vi "Update_FFID_Bkgnd_info.vi"(1 "Specific Bkgnd Meas?":bool, 2 "c^2 (ppm^2)":dbl[](array[numeric]), 3 "C (ppm)":dbl[](array[numeric])) -> ()   [LabVIEW 2015]
uses:
  Controls/Analysis_info_cluster.ctl
  Controls/Inst_type.ctl
  Controls/Instrument_Array.ctl
  Globals/Meas_global.vi
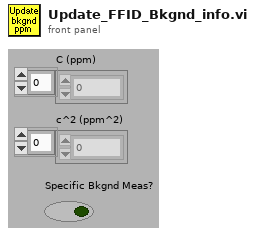
[diagram p1: front panel]
types:
  T1 = cluster{"Weighting":dbl[], "Time (ms)":dbl[], "Voltage":dbl[], "Eng Values":dbl[]}
  T2 = typedef "Analysis_info_cluster.ctl" = cluster{"Colour":u32, "Inst type":T3, "Inst name":string, "Symbol":string, "Code name":string, "Extra Info":string, "Inst Array":T4, "Extra Titles":string[], "Extra Values":string[], "U":dbl, "u^2":dbl, "u^3":dbl, "u^4":dbl, "Skew_u":dbl, "Kurt_u":dbl, "Sd Error in Mean":dbl, "% u'/U":dbl, "X":dbl, "Y":dbl, "Z":dbl, "Timescale integral to 25%":dbl, "Sd Error in Variance":dbl, "Calib File":path, "Calib Constants":dbl[], "Output Position":bool, "Full Stats":bool, "Av Sampling Rate":dbl, "Av No of Samples":dbl, "Total Meas Time (s)":dbl, "ADAM Ch Name":string}
  T3 = typedef "Inst_type.ctl" = enum16{"Propeller anemometer", "Raw voltage", "Pressure Transducer", "Pitot-static tube", "Preston tube", "Hot wire", "Cross wire 1", "Cross wire 2", "Generic Linear", "Generic Polynomial", "Generic BackPoly", "Fast FID", "Thermocouple", "Cold wire", "Pulsed Wire", "LDA Vel", "LDA Tran time", "LDA Arr time", "Microphone"}
  T4 = typedef "Instrument_Array.ctl" = enum16{"PWA", "LDA", "Analogue"}
  T5 = typedef "Time_Trace_Cluster.ctl" = cluster{"Weighting":dbl[], "Time (s)":dbl[], "Voltage":dbl[], "Eng Values":dbl[]}
  T6 = cluster{"Weighting":dbl[], "Time (ms)":dbl[], "Voltage":dbl[], "Eng Values":dbl[]}[]
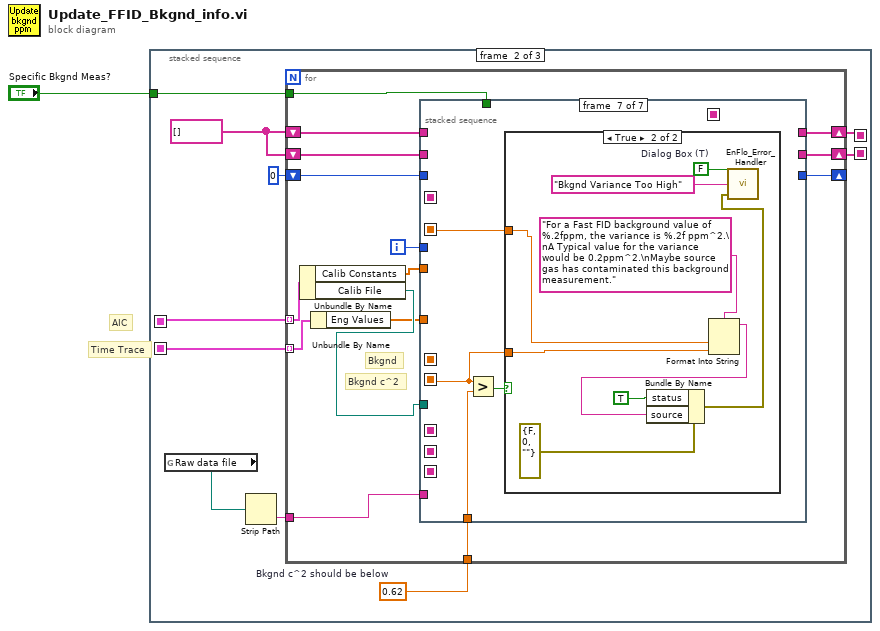
[diagram p0: block diagram]
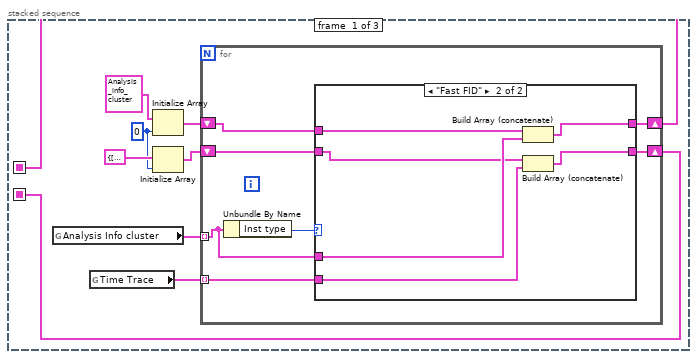
[diagram p2: hidden frame]
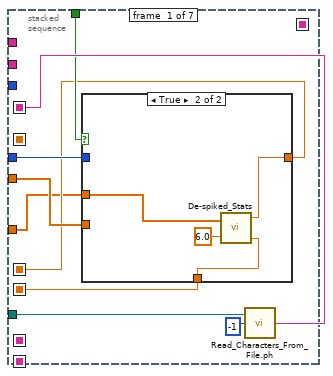
[diagram p4: hidden frame]
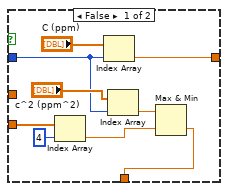
[diagram p5: hidden frame]
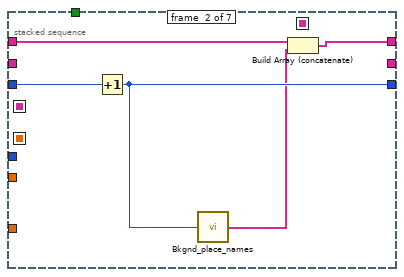
[diagram p6: hidden frame]
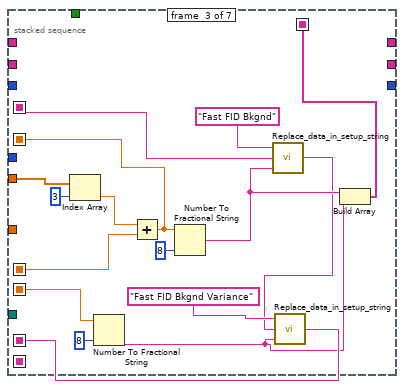
[diagram p7: hidden frame]
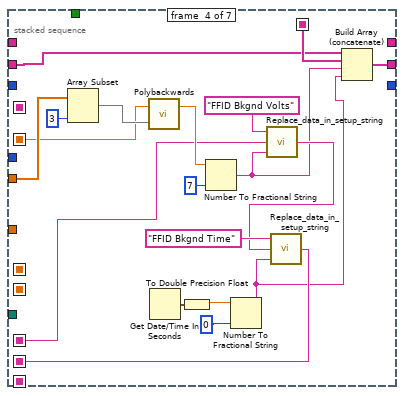
[diagram p8: hidden frame]
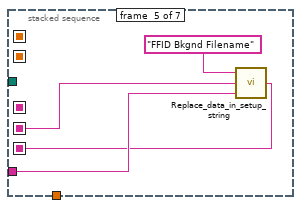
[diagram p9: hidden frame]
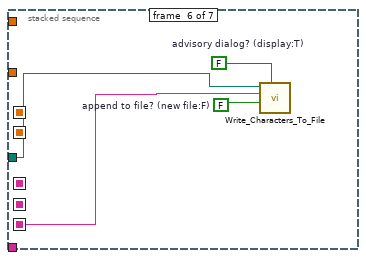
[diagram p10: hidden frame]
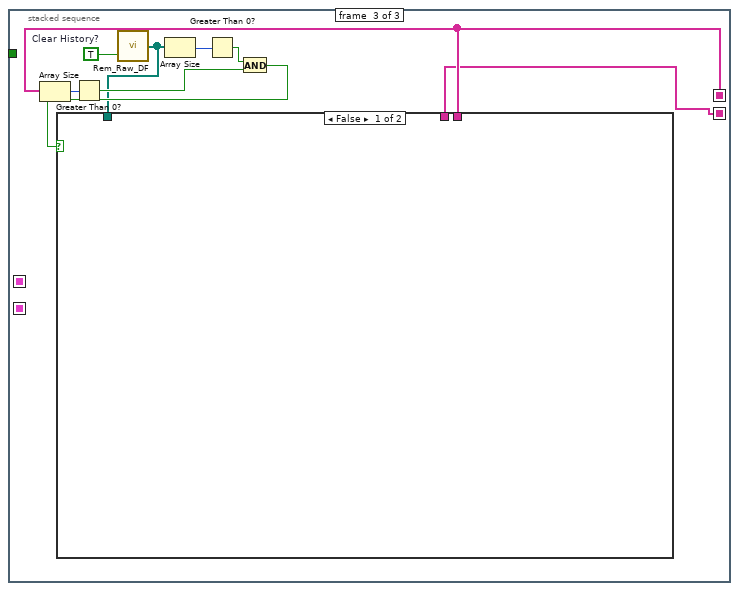
[diagram p12: hidden frame]
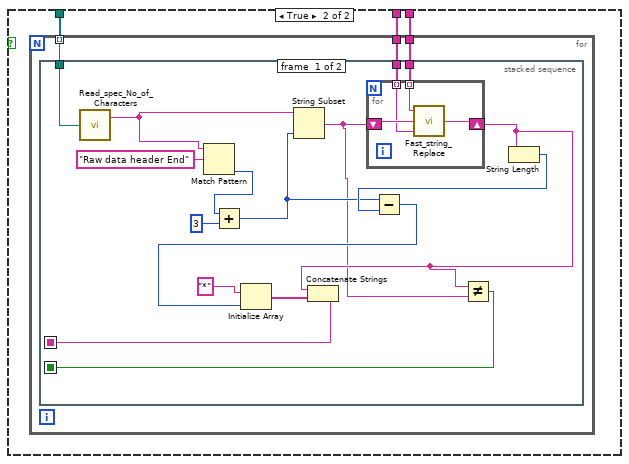
[diagram p13: hidden frame]
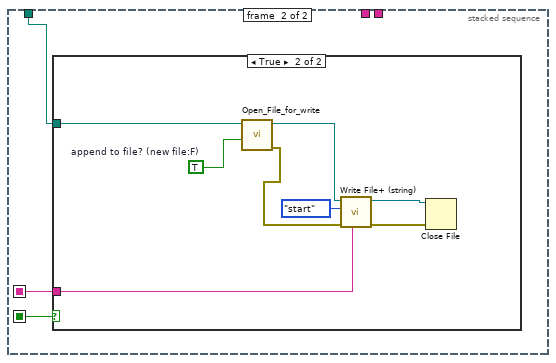
[diagram p14: hidden frame]
diagram:
  # "Time Trace"
  # "AIC"
  n1 = stacked-sequence {
    seq-local: [_ w31 _] -> [_ _ w136]
    seq-local: [_ w30 _] -> [_ _ w135]
    seq-local: [w9 _ _] -> [_ w28 _]
    seq-local: [w2 _ _] -> [_ w26 _]
    tunnel: "Specific Bkgnd Meas?" -> [_ w27 _]
    frame #0 {
      w3 = 0 ("dimension size")
      n2 = global read "Meas_global.vi" "Analysis Info cluster"() -> (w10:T2[])
      n3 = global read "Meas_global.vi" "Time Trace"() -> (w6:T5[])
      n4 = Initialize Array(T2 {"Colour"=0, "Inst type"=enum."Pitot-static tube", "Inst name"="Manometer voltage", "Symbol"="U", "Code name"="", "Extra Info"="U", "Inst Array"=enum."PWA", "Extra Titles"=[], "Extra Values"=[], "U"=0.0, "u^2"=0.0, "u^3"=0.0, "u^4"=0.0, "Skew_u"=0.0, "Kurt_u"=0.0, "Sd Error in Mean"=0.0, "% u'/U"=0.0, "X"=0.0, "Y"=0.0, "Z"=0.0, "Timescale integral to 25%"=0.0, "Sd Error in Variance"=0.0, "Calib File"=path "", "Calib Constants"=[], "Output Position"=FALSE, "Full Stats"=FALSE, "Av Sampling Rate"=0.0, "Av No of Samples"=0.0, "Total Meas Time (s)"=0.0, "ADAM Ch Name"=""} ("Analysis_info_cluster"), w3) -> (w7:T2[])
      n5 = Initialize Array(T1 {"Weighting"=[], "Time (ms)"=[], "Voltage"=[], "Eng Values"=[]} ("Time Trace"), w3) -> (w5:T6)
      n6 = for {
        shift-right: [w15] -> w9
        shift-left: w7 -> [w16]
        tunnel: w10 -> [w14] mode=indexing
        tunnel: w6 -> [w13] mode=indexing
        shift-right: [w11] -> w2
        shift-left: w5 -> [w12]
        n7 = Unbundle By Name(w14) -> ("Inst type"=w17:T3)
        n8 = case shown="\"Fast FID\"" w17 {
          tunnel: w16 -> [w19 w25]
          tunnel: [w19 w23] -> w15
          tunnel: w14 -> [_ w24]
          tunnel: w13 -> [_ w22]
          tunnel: w12 -> [w18 w21]
          tunnel: [w18 w20] -> w11
          frame "Propeller anemometer", Default {
          }
          frame "Fast FID" {
            n9 = Build Array (concatenate)(w25, w24) -> (w23:T2[])
            n10 = Build Array (concatenate)(w21, w22) -> (w20:T5[])
          }
        }
      }
    }
    frame #1 {
      w29 = 0.62  # Bkgnd c^2 should be below
      w32 = string[] []
      n11 = global read "Meas_global.vi" "Raw data file"() -> (w35:path)
      n12 = Strip Path(path=w35) -> (name=w34:string)  [unwired: 1 out]
      n13 = for {
        tunnel: w34 -> [w50]
        shift-right: [w48] -> _
        shift-left: 0 -> [w49]
        shift-right: [w44] -> w30
        shift-left: w32 -> [w45]
        shift-right: [w46] -> w31
        shift-left: w32 -> [w47]
        tunnel: w29 -> [w43]
        tunnel: w28 -> [w40] mode=indexing
        tunnel: w27 -> [w42]
        tunnel: w26 -> [w37] mode=indexing
        i -> [w41]
        # "Bkgnd c^2"
        # "Bkgnd"
        n14 = Unbundle By Name(w40) -> ("Calib Constants"=w39:dbl[], "Calib File"=w38:path)
        n15 = Unbundle By Name(w37) -> ("Eng Values"=w36:dbl[])
        n16 = stacked-sequence {
          seq-local: [w58 _ _ _ _ _ _] -> [_ _ w88 _ _ _ _]
          seq-local: [_ _ w86 _ _ _ _] -> [_ _ _ w101 _ _ _]
          seq-local: [_ _ w84 _ _ _ _] -> [_ _ _ w109 _ _ w124]
          seq-local: [_ _ _ w99 _ _ _] -> [_ _ _ _ w113 _ _]
          seq-local: [_ _ _ _ w114 _ _] -> [_ _ _ _ _ w118 _]
          seq-local: [_ _ w80 _ _ _ _] -> [_ _ _ w98 _ _ _]
          seq-local: [w55 _ _ _ _ _ _] -> [_ _ w79 _ _ _ w123]
          seq-local: [w52 _ _ _ _ _ _] -> [_ _ w78 _ _ _ _]
          tunnel: w39 -> [w54 _ w93 w112 _ _ _]
          tunnel: w38 -> [w57 _ _ _ _ w117 _]
          tunnel: w50 -> [_ _ _ _ w115 _ _]
          tunnel: w49 -> [_ w77 _ _ _ _ _]
          tunnel: [_ w76 _ _ _ _ _] -> w48
          tunnel: w47 -> [_ w74 _ _ _ _ _]
          tunnel: [_ w73 _ _ _ _ _] -> w46
          tunnel: w45 -> [_ _ _ w95 _ _ _]
          tunnel: [_ _ _ w94 _ _ _] -> w44
          tunnel: w43 -> [_ _ _ _ _ _ w121]
          tunnel: w42 -> [w56 _ _ _ _ _ _]
          tunnel: w41 -> [w53 _ _ _ _ _ _]
          tunnel: w36 -> [w51 _ _ _ _ _ _]
          frame #0 {
            n17 = case shown="True" w56 {
              tunnel: [w60 w70] -> w55
              tunnel: w54 -> [w68 _]
              tunnel: w53 -> [w63 _]
              tunnel: [w65 w71] -> w52
              tunnel: w51 -> [_ w69]
              frame False {
                n18 = Index Array(array=w68, index=4) -> (element=w61:dbl)
                n19 = Index Array(array="C (ppm)", index=w63) -> (element=w65:dbl)
                n20 = Index Array(array="c^2 (ppm^2)", index=w63) -> (element=w62:dbl)
                n21 = Max & Min(x=w62, y=w61) -> (min(x,y)=w60:dbl)  [unwired: 1 out]
              }
              frame True {
                n22 = call "De-spiked_Stats.vi"("Raw Signal"=w69, "No of st dev to chop at"=6.0) -> ("mean"=w71:dbl, "variance"=w70:dbl)  [unwired: 1 out]
              }
            }
            n23 = call "Read_Characters_From_File.ph.vi"("file path (dialog if empty)"=w57, "number of characters (all:-1)"=-1) -> ("character string"=w58:string)  [unwired: 7 out]
          }
          frame #1 {
            n24 = Increment(x=w77) -> (x+1=w76:i32)
            n25 = call "Bkgnd_place_names.vi"("Numeric"=w76) -> ("Array"=w75:string[])
            n26 = Build Array (concatenate)(w74, w75) -> (w73:string[])
          }
          frame #2 {
            n27 = Index Array(array=w93, index=3 ("Index")) -> (element=w91:dbl)
            n28 = Number To Fractional String(number=w79, precision (6)=i16 8) -> (F-format string=w81:string)  [unwired: 2 out]
            n29 = Add(x=w91, y=w78) -> (x+y=w84:dbl)
            n30 = Number To Fractional String(number=w84, precision (6)=i16 8) -> (F-format string=w83:string)  [unwired: 2 out]
            n31 = call "Replace_data_in_setup_string.vi"("New data string"=w83, "Input string"=w88, "Variable name"="Fast FID Bkgnd") -> ("Appended string"=w82:string)
            n32 = call "Replace_data_in_setup_string.vi"("New data string"=w81, "Input string"=w82, "Variable name"="Fast FID Bkgnd Variance") -> ("Appended string"=w86:string)
            n33 = Build Array(w83, w81) -> (w80:string[])
          }
          frame #3 {
            n34 = Array Subset(array=w112, length=3 ("index")) -> (w110:dbl[])  [unwired: 1 in]
            n35 = call "Polybackwards.vi"("Coefficients"=w110, "Y input"=w109) -> ("X output"=w108:dbl)  [unwired: 1 out]
            n36 = Get Date/Time In Seconds() -> (seconds since 1Jan1904=w105:timestamp)
            n37 = To Double Precision Float(number=w105) -> (double precision float=w103:dbl)
            n38 = Number To Fractional String(number=w108, precision (6)=i16 7) -> (F-format string=w97:string)  [unwired: 2 out]
            n39 = Number To Fractional String(number=w103, precision (6)=i16 0) -> (F-format string=w96:string)  [unwired: 2 out]
            n40 = call "Replace_data_in_setup_string.vi"("New data string"=w97, "Input string"=w101, "Variable name"="FFID Bkgnd Volts") -> ("Appended string"=w100:string)
            n41 = call "Replace_data_in_setup_string.vi"("New data string"=w96, "Input string"=w100, "Variable name"="FFID Bkgnd Time") -> ("Appended string"=w99:string)
            n42 = Build Array (concatenate)(w95, w98, w97, w96) -> (w94:string[])
          }
          frame #4 {
            n43 = call "Replace_data_in_setup_string.vi"("New data string"=w115, "Input string"=w113, "Variable name"="FFID Bkgnd Filename") -> ("Appended string"=w114:string)
          }
          frame #5 {
            w119 = FALSE  # advisory dialog? (display:T)
            w120 = FALSE  # append to file? (new file:F)
            n44 = call "Write_Characters_To_File.vi"("file path (dialog if empty)"=w117, "advisory dialog? (display:T)"=w119, "character string"=w118, "append to file? (new file:F)"=w120) -> ()  [unwired: 1 in, 4 out]
          }
          frame #6 {
            n45 = Greater?(x=w123, y=w121) -> (0:w122:bool)
            n46 = case shown="True" w122 {
              tunnel: w123 -> [_ w130]
              tunnel: w124 -> [_ w129]
              frame False {
              }
              frame True {
                w125 = FALSE  # Dialog Box (T)
                n47 = Format Into String(format string="For a Fast FID background value of %.2fppm, the variance is %.2f ppm^2.\nA Typical value for the variance would be 0.2ppm^2.\nMaybe source gas has contaminated this background measurement.", w129, w130) -> (resulting string=w127:string)  [unwired: 2 in, 1 out]
                n48 = Bundle By Name(cluster=errorcluster {"status"=FALSE, "code"=0, "source"=""} ("error in (no error)"), "status"=TRUE, "source"=w127) -> (w126:errorcluster)
                n49 = call "EnFlo_Error_Handler.vi"("error in (no error)"=w126, "Error Type"="Bkgnd Variance Too High", "Dialog Box (T)"=w125) -> ()  [unwired: 3 out]
              }
            }
          }
        }
      }
    }
    frame #2 {
      w134 = TRUE  # Clear History?
      n50 = Array Size(array=w136) -> (size(s)=w141:i32)
      n51 = Greater Than 0?(x=w141) -> (x > 0?=w139:bool)
      n52 = call "Rem_Raw_DF.vi"("Clear History?"=w134) -> ("List of Filenames"=w137:path[])  [unwired: 1 in]
      n53 = Array Size(array=w137) -> (size(s)=w142:i32)
      n54 = Greater Than 0?(x=w142) -> (x > 0?=w140:bool)
      n55 = And(x=w140, y=w139) -> (x .and. y?=w138:bool)
      n56 = case shown="False" w138 {
        tunnel: w137 -> [_ w145]
        tunnel: w136 -> [_ w144]
        tunnel: w135 -> [_ w143]
        frame False {
        }
        frame True {
          n57 = for {
            tunnel: w145 -> [w146] mode=indexing
            tunnel: w144 -> [w148]
            tunnel: w143 -> [w147]
            n58 = stacked-sequence {
              seq-local: [w152 _] -> [_ w170]
              seq-local: [w150 _] -> [_ w169]
              tunnel: w148 -> [w160 _]
              tunnel: w147 -> [w159 _]
              tunnel: w146 -> [w153 w171]
              frame #0 {
                n59 = call "Read_spec_No_of_Characters.vi"("Filename"=w153) -> ("character string"=w161:string)  [unwired: 1 out]
                n60 = Match Pattern(string=w161, regular expression="Raw data header End") -> (offset past match=w163:i32)  [unwired: 4 out]
                n61 = Add(x=w163, y=3) -> (x+y=w157:i32)
                n62 = String Subset(string=w161, length (rest)=w157) -> (substring=w149:string)  [unwired: 1 out]
                n63 = for {
                  shift-right: [w167] -> w151
                  shift-left: w149 -> [w168]
                  tunnel: w160 -> [w166] mode=indexing
                  tunnel: w159 -> [w165] mode=indexing
                  n64 = call "Fast_string_Replace.vi"("Replace match with:"=w165, "Input String"=w168, "regular expression"=w166) -> ("Output String"=w167:string)  [unwired: 2 out]
                }
                n65 = Not Equal?(x=w151, y=w149) -> (x != y?=w150:bool)
                n66 = String Length(string=w151) -> (length=w158:i32)
                n67 = Subtract(x=w157, y=w158) -> (x-y=w155:i32)
                n68 = Initialize Array("*", w155) -> (w154:string[])
                n69 = Concatenate Strings(w151, w154) -> (w152:string)
              }
              frame #1 {
                n70 = case shown="True" w169 {
                  tunnel: w171 -> [_ w179]
                  tunnel: w170 -> [_ w172]
                  frame False {
                  }
                  frame True {
                    w178 = TRUE  # append to file? (new file:F)
                    n71 = call "Open_File_for_write.vi"("append to file? (new file:F)"=w178, "file path"=w179) -> ("error out"=w175:errorcluster, "refnum"=w176:refnum<file>)  [unwired: 1 in, 7 out]
                    n72 = call <vilib>:"Write File+ (string).vi"("string"=w172, "error in (no error)"=w175, "pos mode (rel. to end:1)"=enum16{"start", "end", "current"}."start", "refnum"=w176) -> ("error out"=w173:errorcluster, "dup refnum"=w174:refnum<file>)  [unwired: 1 in, 3 out]
                    n73 = Close File(refnum=w174, error in=w173) -> ()  [unwired: 2 out]
                  }
                }
              }
            }
          }
        }
      }
    }
  }
